vi "UI.vi"(0 "reference in":refnum<class "GUI Work Windows.lvclass">, 5 "error in (no error)":errorcluster) -> (14 "reference out":refnum<class "GUI Work Windows.lvclass">, 19 "error out":errorcluster)   [LabVIEW 2019, in "GUI Work Windows.lvclass"]
uses:
  GUI Work Windows.lvclass
  D:/GIT H4000/H4000/src/GUI_class/GUI.lvclass
  TypeDef/Data Stand.ctl
  TypeDef/Mode.ctl
  TypeDef/ExecuteStepState.ctl
  TypeDef/Direction.ctl
  Modbus_class/STS REG.ctl
  TypeDef/SP_TYPE.ctl
  TypeDef/State 44-1-2.ctl
  Modbus_class/CMD REG.ctl
  GUI_class/GUI.lvclass/GUI.ctl
  TypeDef/AI_Data_Array.ctl
  TypeDef/AI_Data.ctl
  TypeDef/AI Statistics Data.ctl
  FPGA/TypeDef/AI index.ctl
  SV_Wrap/SharedVariableWrapper.lvclass/SharedVariableWrapper.ctl
  Logger_class/Current Alarms.ctl
  Logger_class/EventData.ctl
  TypeDef/AlarmType.ctl
  MessageAMC_class/MessageAMC.lvclass
  D:/GIT H4000/H4000/src/MessageInterface_class/MessageInterface.lvclass
  f117a657-4c7e-47d8-9c03-ebf14d957611.vi
  1dd7af2e-2118-4c7c-a33f-1a736c63832f.vi
  8ac79095-62ac-4481-ab6e-8384228cdb70.vi
  41a135e7-8ee8-4611-b48a-c3c60048d180.vi
  6e9eca7a-d5d6-4f73-afb0-1afe8d30e139.vi
  a088a5f2-3759-4c3f-ba66-888ae32085c6.vi
  020c85a8-0765-46a5-946e-679e8cc30ba7.vi
  a65858e0-b92e-4e89-be62-7fc9634f1b2d.vi
  b775c166-e071-486c-b96e-0b96b0641e47.vi
  bf4e41d3-c56e-4c10-8d22-db1e327fdeb2.vi
  f5c6e87b-12af-4f11-98e9-46c3725dc062.vi
  c40ac8ee-f23a-4eac-9387-617ed5b7c06a.vi
  4e247ec6-9307-4091-8dab-29632f0d07b9.vi
  6be4fd1c-314b-4f5a-9423-f44751c79fde.vi
  010ce43b-0ee2-4248-bca4-f765867da5e8.vi
  GUI_class/Set Win State.vi
  GUI_class/protected/GetSheredData.vi
  8ac79095-62ac-4481-ab6e-8384228cdb70.vi/e1ff1487-cd56-43d2-a3a5-d033708db06e.vi
  SV_Wrap/Write Var Info.vi
  SV_Wrap/Read Var Info.vi
  41a135e7-8ee8-4611-b48a-c3c60048d180.vi/1efd96e0-8378-4666-9377-02721ba78358.vi
  6e9eca7a-d5d6-4f73-afb0-1afe8d30e139.vi/bae99f4a-ec10-4ec0-96ec-6d26d63f25ad.vi
  a088a5f2-3759-4c3f-ba66-888ae32085c6.vi/8d9527f5-1861-4624-9257-997a85ef616e.vi
  020c85a8-0765-46a5-946e-679e8cc30ba7.vi/7d84ca54-f83c-4ce5-86c1-7a192ad6100d.vi
  a65858e0-b92e-4e89-be62-7fc9634f1b2d.vi/5b02730d-42c6-4a71-85e1-f046919fac21.vi
  SV_Wrap/Read connection str.vi
  <userlib>/_OpenG.lib/time/time.llb/Tick Count (ms)__ogtk.vi
  GUI_class/GUI.lvclass
  SV_Wrap/SharedVariableWrapper.lvclass
  MessageInterface_class/MessageInterface.lvclass
panel:
  in  "hold":bool caption="Разрешить удержание"
  out "duration":i64
  out "delta dut 2":dbl caption="Погрешность [%]" format="%.1g"
  out "delta dut":dbl caption="Погрешность [%]" format="%.1g"
  in  "buret time":u16 caption="Время открытия бюретки [сек]"
  in  "nitro":bool caption="Азот"
  in  "burette":bool caption="Бюретка"
  in  "sp chamber":dbl caption="Уставка камера [МПа]"
  in  "sp dut":dbl caption="Уставка образец [МПа]"
  in  "CMD REG":T1
  out "leak":dbl(graph) caption="Давление датчик утечек [МПа]"
  out "data out":T2={"CommCounter"=0, "BeginFilingLevel"=0.0, "SP DUT"=0.0, "SP CHAMBER"=0.0, "Mode"=enum."IDLE", "ExecuteStepState"=enum."Init", "Direction"=enum."DUT", "Direction Filling"=enum."DUT", "STS"={"IDLE"=FALSE, "RYADY"=FALSE, "STEP"=FALSE, "ALARM"=FALSE, "WARNING"=FALSE, "REMOTE"=FALSE, "SP_EXEC_DONE_DUT"=FALSE, "SP_EXEC_DONE_CHAMBER"=FALSE, "FILING_DONE_DUT"=FALSE, "FILING_DONE_CHAMBER"=FALSE, "BURETE_STATE"=FALSE}, "SP_TYPE_DUT"=enum."ZIRO", "SP_TYPE_CHAMBER"=enum."ZIRO", "New Step"=FALSE, "BURETE_TIME"=0, "With BURETE"=FALSE, "With Nitro"=FALSE, "State 44-1-2"=enum."Init", "Measure leak"=FALSE, "hold"=FALSE}
  in  "clear chart":bool
  in  "Multicolumn Listbox":i32(listbox)=-1
  out "error":bool caption="Подключение"
  out "chmbr":T9(graph) caption="Давление камера [МПа]"
  out "dut":T9(graph) caption="Давление образец [МПа]"
  in  "remote":bool caption="Разрешить внешнее управление"
  in  "stop":bool
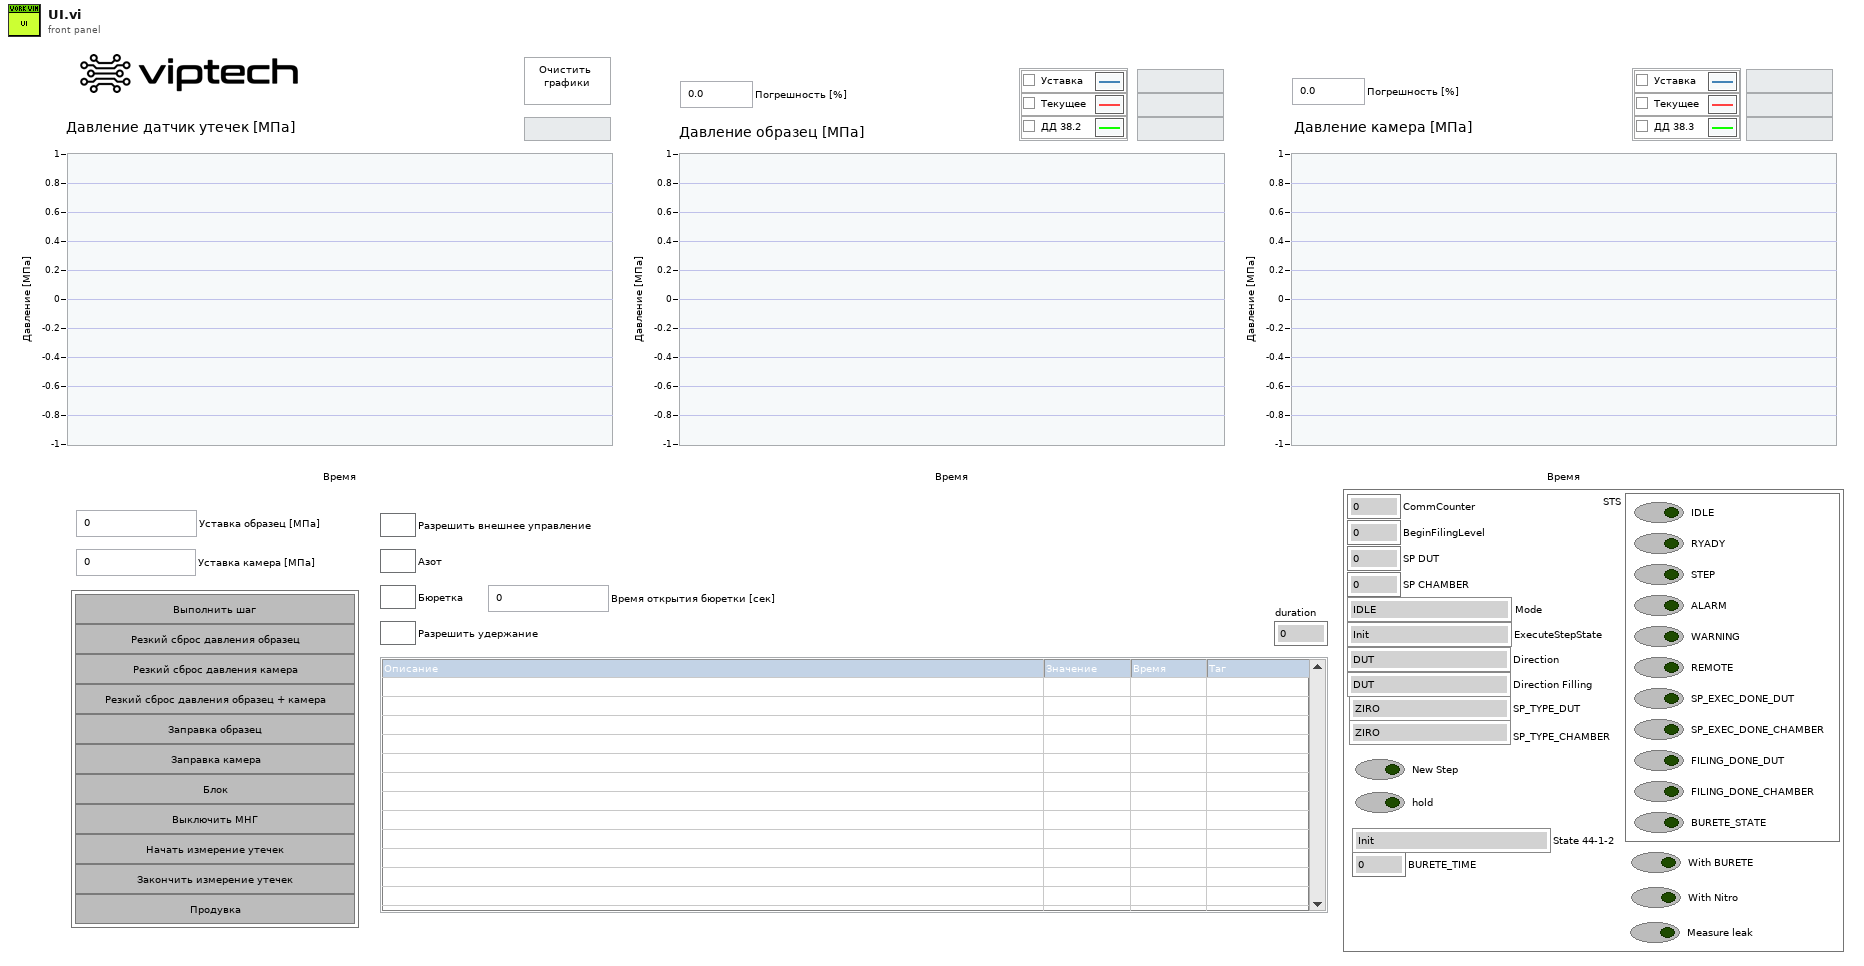
[diagram p1: front panel]
types:
  T1 = typedef "CMD REG.ctl" = cluster{"EXECUTE_SP":bool, "ALARM_PRESS_DOWN_DUT":bool, "ALARM_PRESS_DOWN_CHAMBER":bool, "ALARM_PRESS_DOWN_DUT_CHAMBER":bool, "FILING_DUT":bool, "FILING_CHAMBER":bool, "BLOCK":bool, "PUMP_STATION_OFF":bool, "Leak start":bool, "Leak stop":bool, "Drain":bool}
  T2 = typedef "Data Stand.ctl" = cluster{"CommCounter":u64, "BeginFilingLevel":dbl, "SP DUT":dbl, "SP CHAMBER":dbl, "Mode":T3, "ExecuteStepState":T4, "Direction":T5, "Direction Filling":T5, "STS":T6, "SP_TYPE_DUT":T7, "SP_TYPE_CHAMBER":T7, "New Step":bool, "BURETE_TIME":u16, "With BURETE":bool, "With Nitro":bool, "State 44-1-2":T8, "Measure leak":bool, "hold":bool}
  T3 = typedef "Mode.ctl" = enum16{"IDLE", "FILLING", "EXECUTE_SP", "DRAIN"}
  T4 = typedef "ExecuteStepState.ctl" = enum16{"Init", "Set: Backpressure ", "Preload: HI", "Set: HI", "Maintenance: HI", "Down: Pressure", "BLOCK"}
  T5 = typedef "Direction.ctl" = enum8{"DUT", "Chamber"}
  T6 = typedef "STS REG.ctl" = cluster{"IDLE":bool, "RYADY":bool, "STEP":bool, "ALARM":bool, "WARNING":bool, "REMOTE":bool, "SP_EXEC_DONE_DUT":bool, "SP_EXEC_DONE_CHAMBER":bool, "FILING_DONE_DUT":bool, "FILING_DONE_CHAMBER":bool, "BURETE_STATE":bool}
  T7 = typedef "SP_TYPE.ctl" = enum16{"ERROR", "ZIRO", "BASE", "SP"}
  T8 = typedef "State 44-1-2.ctl" = enum16{"Init", "Idle", "Wait", "Open 44-1", "Open 44-2", "Close 44-1", "Close 44-2"}
  T9 = cluster{"Pressure SP":dbl, "scl mean 1Hz":dbl, "scl mean 1Hz":dbl}
  T10 = enum32{"Invalid", "Standard", "Closed", "Hidden", "Minimized", "Maximized"}
  T11 = enum32{"invalid app kind", "Development System", "Run Time System", "Student Edition", "Embedded LabVIEW", "Evaluation", "Custom"}
  T12 = typedef "SharedVariableWrapper.lvclass/Config.ctl" = cluster{"connection str":string, "timeout":dbl, "ip":string}
  T13 = cluster{"Core":cluster{"Current VI Reference":refnum<vi>, "Close Panel on Exit?":bool}, "amc":refnum<class "MessageAMC.lvclass">}
  T14 = cluster{"Current VI Reference":refnum<vi>, "Close Panel on Exit?":bool}
  T15 = typedef "AI_Data_Array.ctl" = T16[]
  T16 = typedef "AI_Data.ctl" = cluster{"Stat Data":T17, "OutOfRangeMax":bool, "OutOfRangeMin":bool, "HIHI":bool, "HI":bool, "LO":bool, "LOLO":bool}
  T17 = typedef "AI Statistics Data.ctl" = cluster{"raw mean":dbl, "scl mean":dbl, "raw mean 1Hz":dbl, "scl mean 1Hz":dbl}
  T18 = typedef "Current Alarms.ctl" = cluster{"alarms":T19[]}
  T19 = typedef "EventData.ctl" = cluster{"obj_tag":string, "event_tag":string, "Description":string, "ALARM TYPE":T20, "Value DBL":dbl, "Value INT":i32, "Value STR":string, "Time Stamp":timestamp}
  T20 = typedef "AlarmType.ctl" = enum16{"Normal", "Warning", "Alarm"}
  T21 = typedef "AI index.ctl" = u8
  T22 = cluster{"SP DUT":dbl, "scl mean 1Hz":dbl, "scl mean 1Hz":dbl}
  T23 = cluster{"SP CHAMBER":dbl, "scl mean 1Hz":dbl, "scl mean 1Hz":dbl}
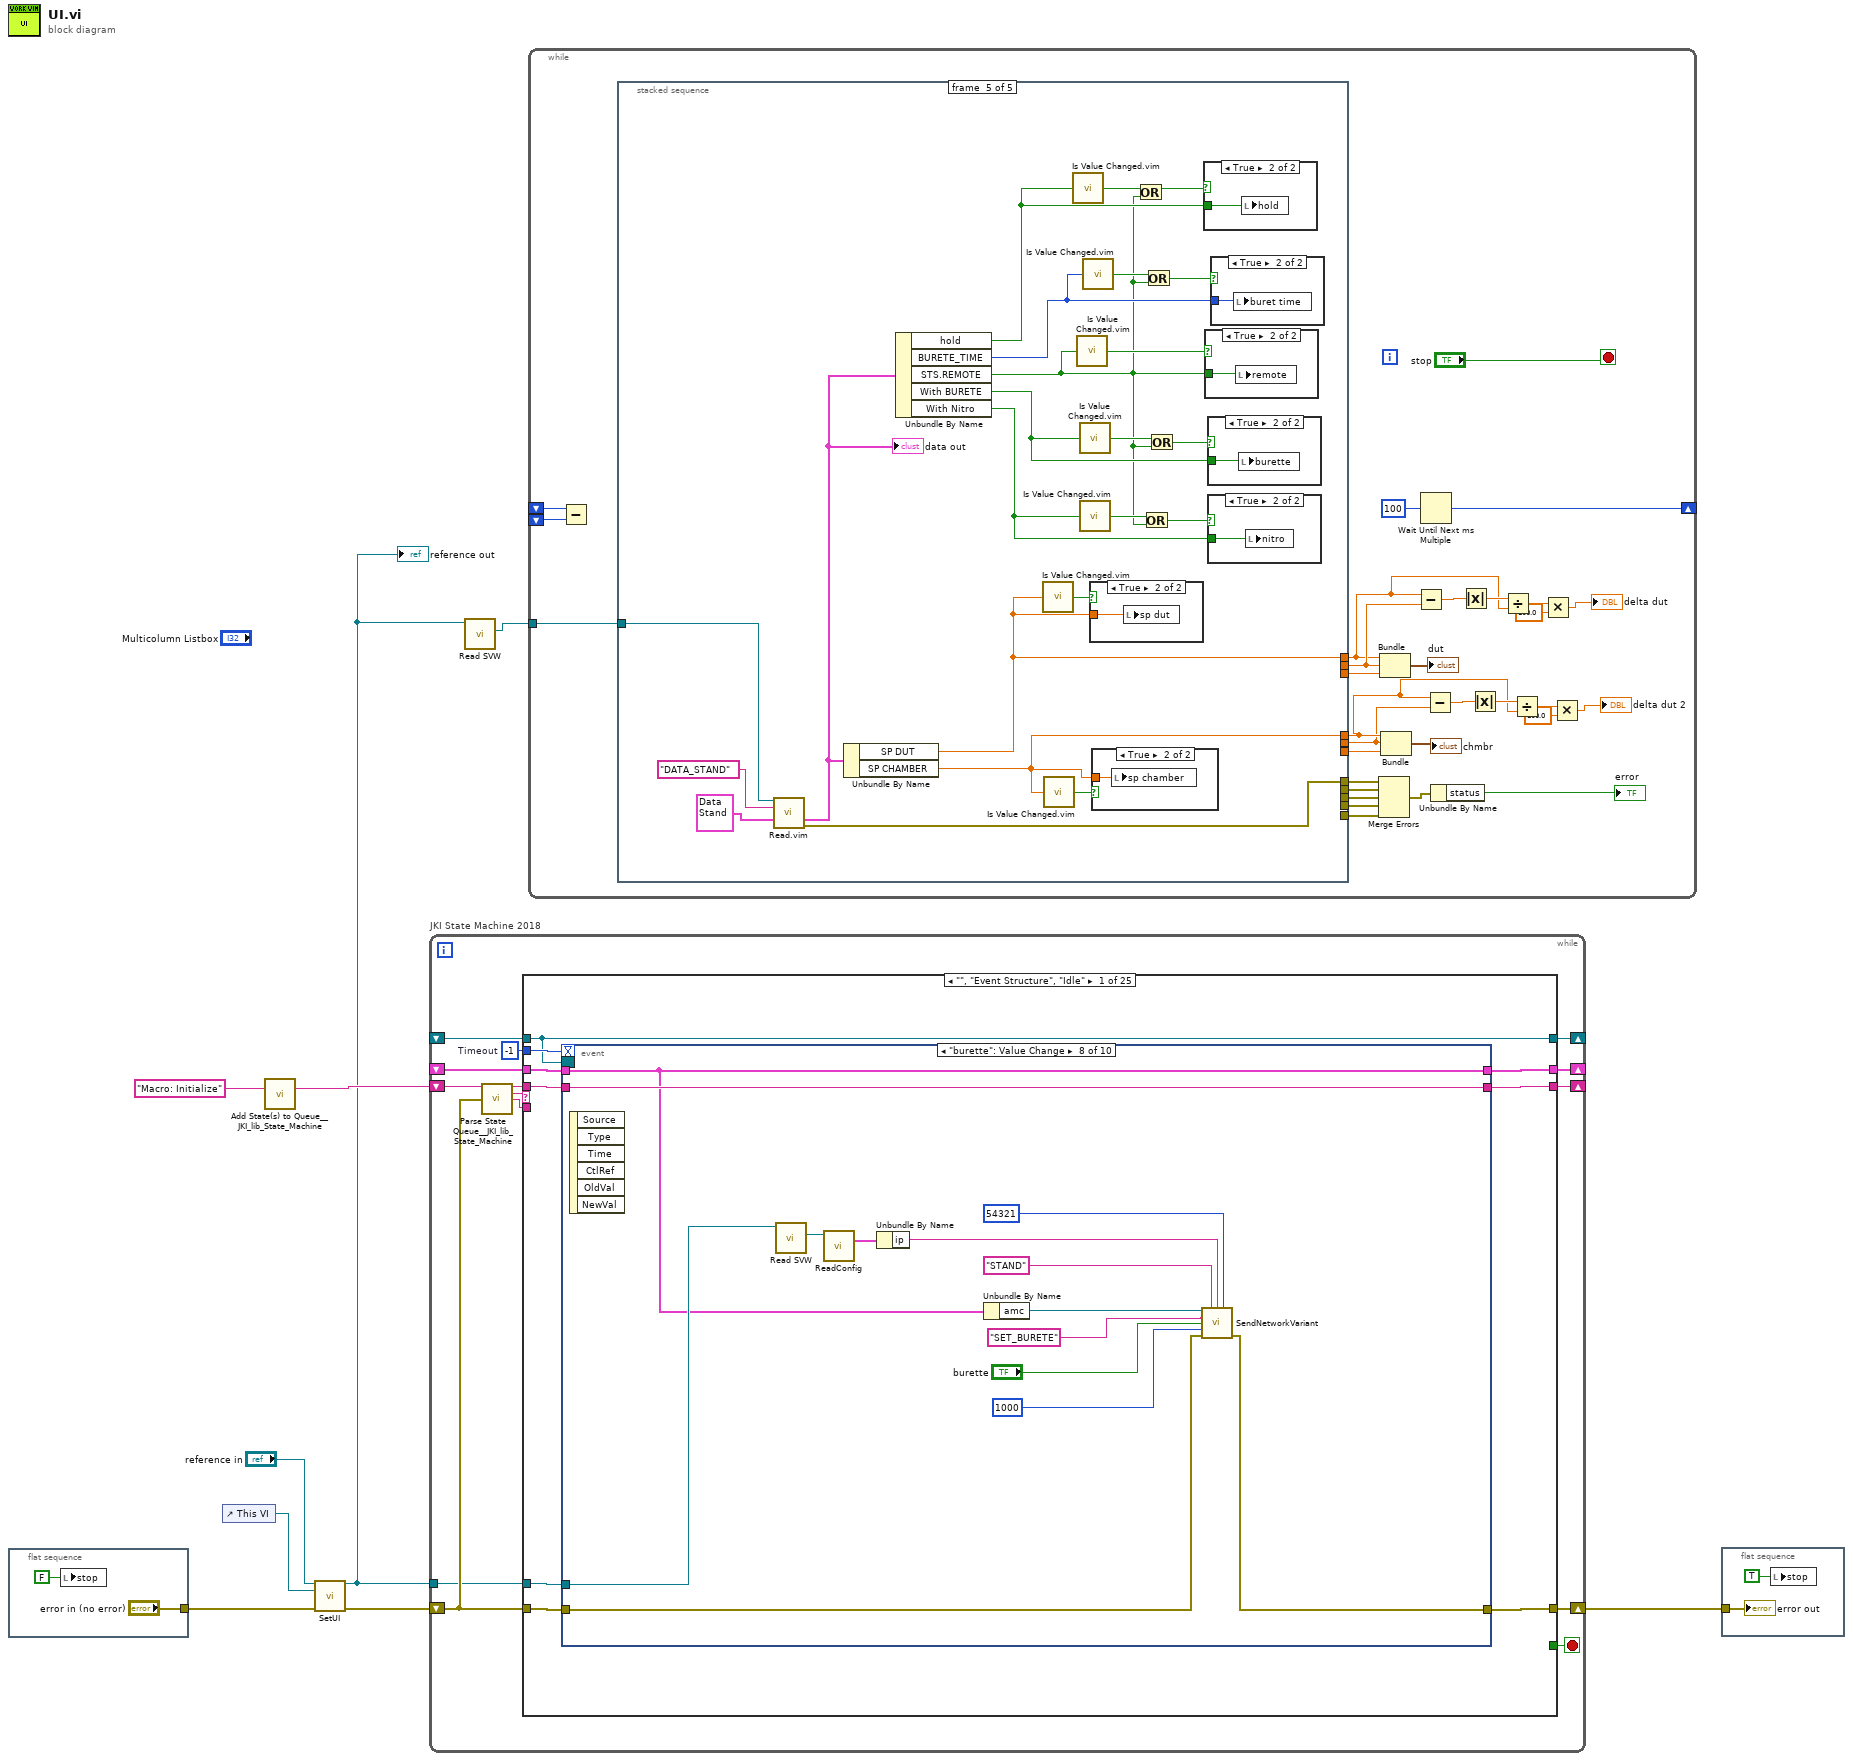
[diagram p0: block diagram]
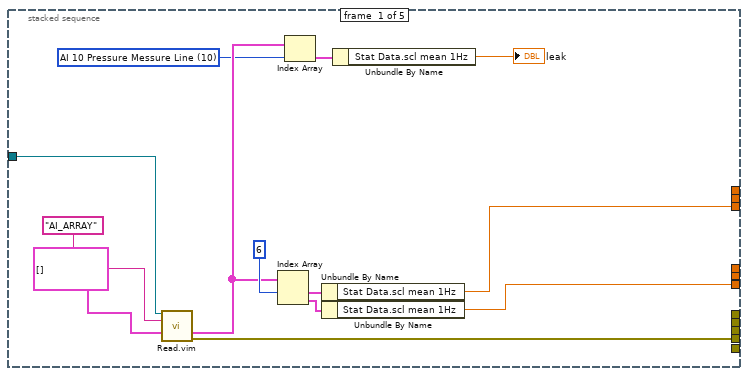
[diagram p2: hidden frame]
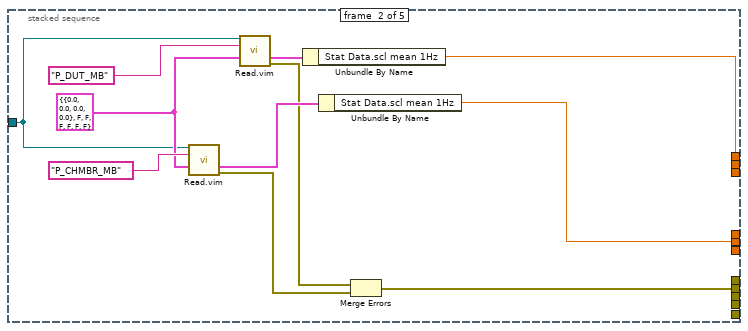
[diagram p3: hidden frame]
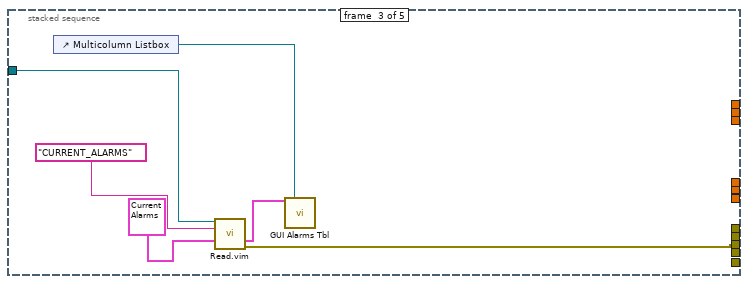
[diagram p4: hidden frame]
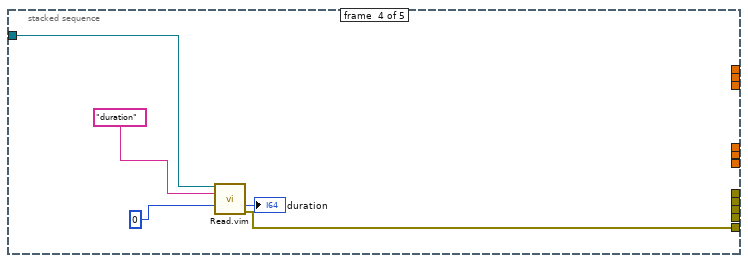
[diagram p5: hidden frame]
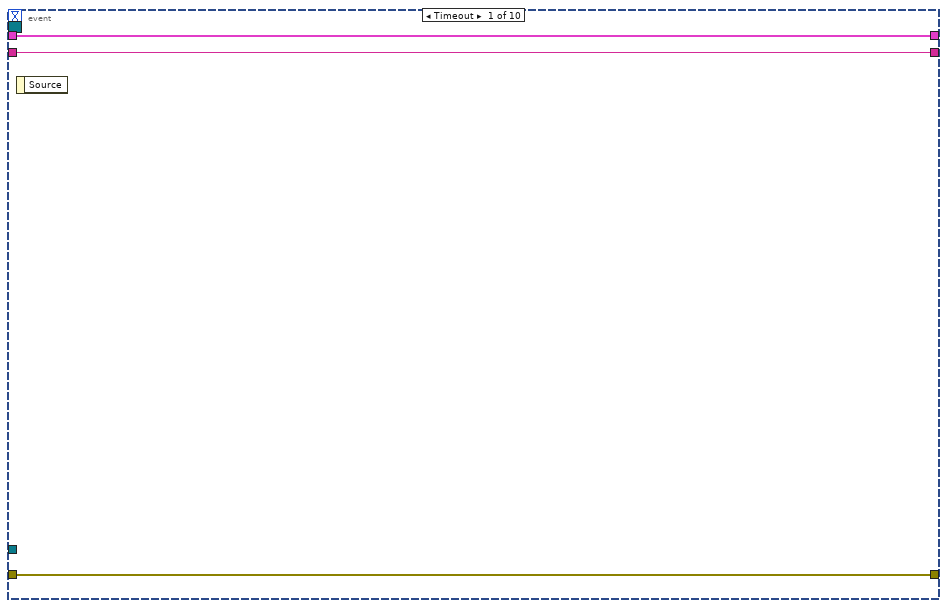
[diagram p13: hidden frame]
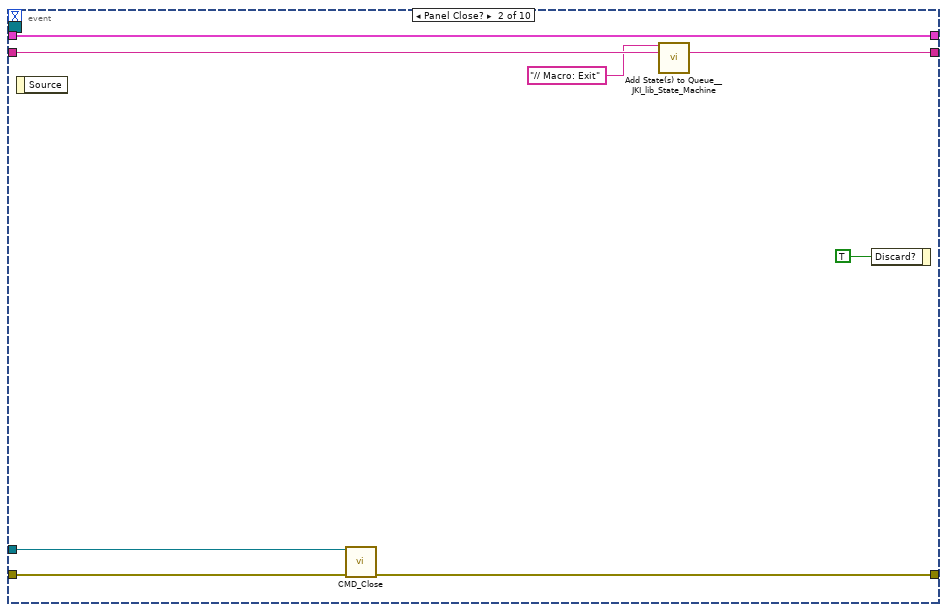
[diagram p14: hidden frame]
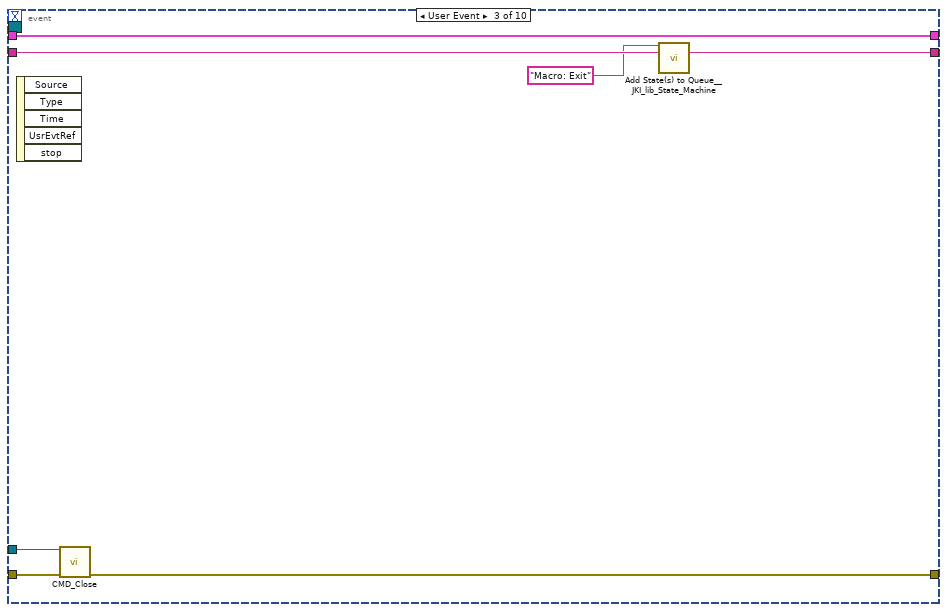
[diagram p15: hidden frame]
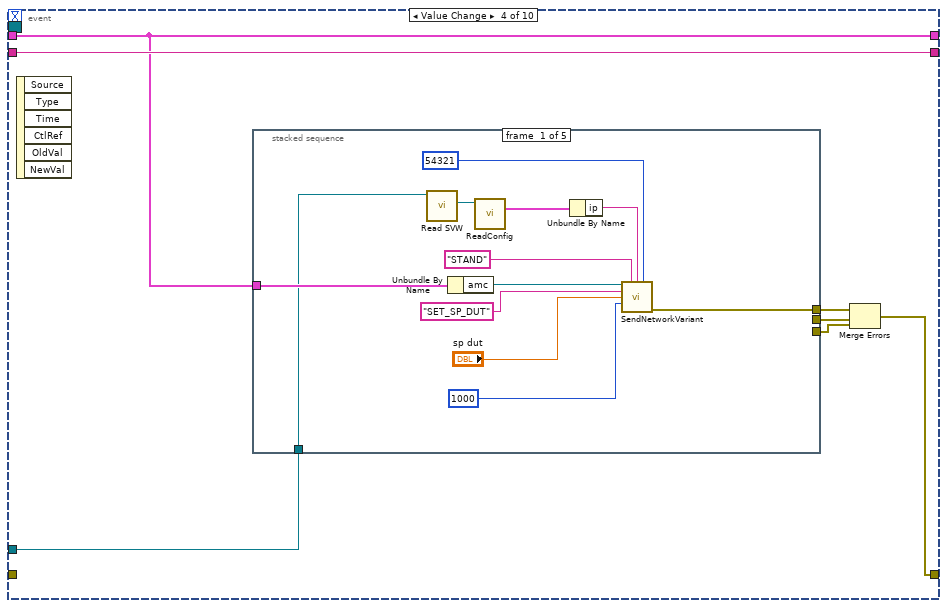
[diagram p16: hidden frame]
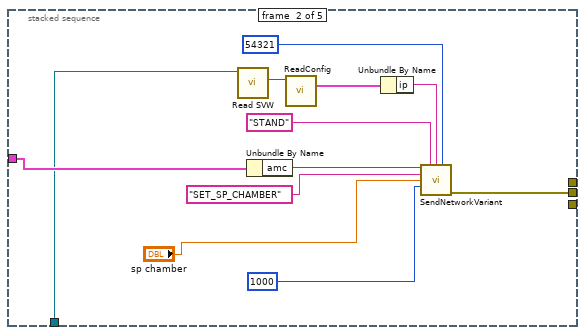
[diagram p17: hidden frame]
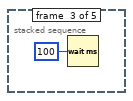
[diagram p18: hidden frame]
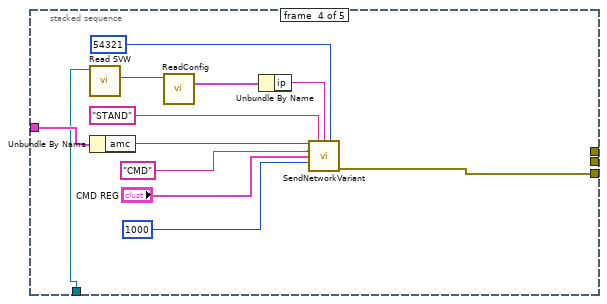
[diagram p19: hidden frame]
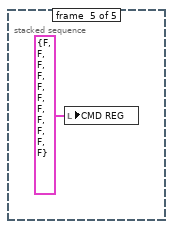
[diagram p20: hidden frame]
diagram:
  n1 = flat-sequence {
    tunnel: ["error in (no error)"] -> w6
    frame #0 {
      n2 = local write "stop"(FALSE ("stop")) -> ()
    }
  }
  n3 = control-ref of="This VI"() -> (w4:refnum<vi>)
  n4 = call <vilib>:"Add State(s) to Queue__JKI_lib_State_Machine.vi"("State(s) in (\"\")"="Macro: Initialize") -> ("States Out"=w9:string)  [unwired: 14 in]
  n5 = call "SetUI.vi"("reference in"="reference in", "UI VI"=w4, "error in (no error)"=w6) -> ("reference out"=w2:refnum<class "GUI Work Windows.lvclass">, "error out"=w3:errorcluster)  [unwired: 11 in]
  "reference out" <- w2
  n6 = while "JKI State Machine 2018" {
    shift-right: [w18] -> _
    shift-left: _ -> [w17]
    shift-right: [w21] -> w7
    shift-left: w3 -> [w15]
    shift-right: [w20] -> _
    shift-left: w9 -> [w22]
    tunnel: w2 -> [w14]
    shift-right: [w13] -> _
    shift-left: _ -> [w12]
    stop <- w19 stop-if-true
    w16 = -1  # Timeout
    n7 = call <vilib>:"Parse State Queue__JKI_lib_State_Machine.vi"("State Queue"=w22, "Error In (no error)"=w15) -> ("Remaining States"=w24:string, "Current State"=w25:string, "Arguments"=w23:string)  [unwired: 11 in]
    n8 = case shown="\"\", \"Event Structure\", \"Idle\"" w25 {
      selector: w25 -> [_ _ w186 _ _ _ _ _ _ _ _ _ _ _ _ _ _ _ _ _ _ _ _ _ _]
      tunnel: w24 -> [w34 w184 w190 w210 w217 w225 w230 w239 w246 w251 w258 w264 w269 w273 w280 w292 w362 w368 w374 w386 w390 w391 w400 w404 w406]
      tunnel: w23 -> [_ _ _ _ _ _ _ _ _ _ _ _ _ _ w275 w286 _ _ _ _ _ _ _ _ _]
      tunnel: w17 -> [w32 w181 w188 w203 w214 w220 w227 _ w241 w248 w257 w262 w266 w272 w278 w288 w359 w365 w371 w383 w388 w393 w398 w401 w405]
      tunnel: [w31 w182 w192 w207 errorcluster {"status"=FALSE, "code"=0, "source"=""} ("error out") w223 w228 w232 w242 w249 w255 w259 w267 w271 w276 w289 w360 w366 w372 w384 w389 w394 w397 w402 w408] -> w21
      tunnel: w15 -> [w30 w182 w191 w207 w213 w223 w228 w233 w243 w249 w254 w260 w267 w271 w277 w290 w360 w366 w372 w384 w389 w394 w397 w402 w408]
      tunnel: [w33 w183 w189 w209 w216 w224 w229 w239 w245 w250 w258 w263 w268 w273 w279 w291 w361 w367 w373 w385 w390 w392 w400 w404 w406] -> w20
      tunnel: [_ _ _ _ _ TRUE _ _ _ _ _ _ _ _ _ _ _ _ _ _ _ _ _ _ _] -> w19
      tunnel: [w29 w181 w188 w208 w214 w220 w227 w238 w241 w248 w257 w262 w266 w272 w278 w288 w359 w365 w371 w383 w388 w393 w398 w401 w405] -> w18
      tunnel: w16 -> [w28 _ _ _ _ _ _ _ _ _ _ _ _ _ _ _ _ _ _ _ _ _ _ _ _]
      tunnel: w14 -> [w27 _ _ _ _ _ _ _ _ _ w253 _ _ _ _ _ _ _ _ _ _ w395 _ _ _]
      tunnel: [w26 w180 w185 w197 w211 w221 w226 w236 w240 w247 w256 w261 w265 w270 w274 w285 w358 w363 w369 w376 w387 w396 w399 w403 w407] -> w13
      tunnel: w12 -> [w26 w180 w185 w197 w211 w221 w226 w236 w240 w247 _ w261 w265 w270 w274 w285 w358 w363 w369 w376 w387 w396 w399 w403 w407]
      frame "", "Event Structure", "Idle" {
        n9 = event shown="[7] \"burette\": Value Change" {
          selector: w26 -> [_ _ _ _ _ _ _ _ _ _]
          dyn-events: _ -> [_ _ _ _ _ _ _ _ _ _]
          timeout: w28 -> [_ _ _ _ _ _ _ _ _ _]
          tunnel: w34 -> [w37 w45 w52 w59 w106 w123 w137 w151 w165 w179]
          tunnel: [w37 w44 w51 w59 w106 w123 w137 w151 w165 w179] -> w33
          tunnel: w32 -> [w35 w43 w50 w58 w105 w118 w132 w146 w160 w174]
          tunnel: [w36 w38 w46 w53 w99 w111 w125 w139 w153 w167] -> w31
          tunnel: w30 -> [w36 w39 w47 _ w104 w112 w126 w140 w154 w168]
          tunnel: [w35 w43 w50 w58 w105 w118 w132 w146 w160 w174] -> w29
          tunnel: w27 -> [_ w40 w48 w57 _ w119 w133 w147 w161 w175]
          event Timeout {
            n10 = event-data() -> ()  [unwired: 1 in, 1 out]
          }
          event Panel Close? {
            n11 = event-data() -> ()  [unwired: 1 in, 1 out]
            n12 = call "CMD_Close.vi"("reference in"=w40, "error in (no error)"=w39) -> ("error out"=w38:errorcluster)  [unwired: 12 in, 1 out]
            n13 = call <vilib>:"Add State(s) to Queue__JKI_lib_State_Machine.vi"("State(s) in Front (\"\")"="// Macro: Exit", "State(s) in (\"\")"=w45) -> ("States Out"=w44:string)  [unwired: 13 in]
            n14 = event-data("Discard?"=TRUE) -> ()  [unwired: 1 in, 1 out]
          }
          event User Event {
            n15 = event-data() -> ()  [unwired: 1 in, 5 out]
            n16 = call "CMD_Close.vi"("reference in"=w48, "error in (no error)"=w47) -> ("error out"=w46:errorcluster)  [unwired: 12 in, 1 out]
            n17 = call <vilib>:"Add State(s) to Queue__JKI_lib_State_Machine.vi"("State(s) in Front (\"\")"="Macro: Exit", "State(s) in (\"\")"=w52) -> ("States Out"=w51:string)  [unwired: 13 in]
          }
          event Value Change {
            n18 = event-data() -> ()  [unwired: 1 in, 6 out]
            n19 = stacked-sequence {
              tunnel: w58 -> [w63 w74 _ w87 _]
              tunnel: w57 -> [w62 w73 _ w85 _]
              tunnel: [w61 _ _ _ _] -> w54
              tunnel: [_ w72 _ _ _] -> w55
              tunnel: [_ _ _ w88 _] -> w56
              frame #0 {
                n20 = call "Read SVW.vi"("GUI in"=w62) -> ("SharedVariableWrapper.lvclass"=w68:refnum<class "SharedVariableWrapper.lvclass">)  [unwired: 10 in]
                n21 = Unbundle By Name(w63) -> ("amc"=w60:refnum<class "MessageAMC.lvclass">)
                n22 = call "ReadConfig.vi"("SharedVariableWrapper in"=w68) -> ("config"=w69:T12)  [unwired: 12 in, 2 out]
                n23 = Unbundle By Name(w69) -> ("ip"=w70:string)
                n24 = call "SendNetworkVariant.vi"("reference in"=w60, "receiver process"="STAND", "receiver host"=w70, "receiver port (0)"=u16 54321, "name"="SET_SP_DUT", "data"="sp dut", "timeout (25000 ms)"=1000) -> ("error out"=w61:errorcluster)  [unwired: 6 in, 2 out]
              }
              frame #1 {
                n25 = call "Read SVW.vi"("GUI in"=w73) -> ("SharedVariableWrapper.lvclass"=w79:refnum<class "SharedVariableWrapper.lvclass">)  [unwired: 10 in]
                n26 = Unbundle By Name(w74) -> ("amc"=w82:refnum<class "MessageAMC.lvclass">)
                n27 = call "ReadConfig.vi"("SharedVariableWrapper in"=w79) -> ("config"=w80:T12)  [unwired: 12 in, 2 out]
                n28 = Unbundle By Name(w80) -> ("ip"=w81:string)
                n29 = call "SendNetworkVariant.vi"("reference in"=w82, "receiver process"="STAND", "receiver host"=w81, "receiver port (0)"=u16 54321, "name"="SET_SP_CHAMBER", "data"="sp chamber", "timeout (25000 ms)"=1000) -> ("error out"=w72:errorcluster)  [unwired: 6 in, 2 out]
              }
              frame #2 {
                n30 = Wait (ms)(milliseconds to wait=u32 100) -> ()  [unwired: 1 out]
              }
              frame #3 {
                n31 = call "Read SVW.vi"("GUI in"=w85) -> ("SharedVariableWrapper.lvclass"=w96:refnum<class "SharedVariableWrapper.lvclass">)  [unwired: 10 in]
                n32 = Unbundle By Name(w87) -> ("amc"=w86:refnum<class "MessageAMC.lvclass">)
                n33 = call "ReadConfig.vi"("SharedVariableWrapper in"=w96) -> ("config"=w95:T12)  [unwired: 12 in, 2 out]
                n34 = Unbundle By Name(w95) -> ("ip"=w94:string)
                n35 = call "SendNetworkVariant.vi"("reference in"=w86, "receiver process"="STAND", "receiver host"=w94, "receiver port (0)"=u16 54321, "name"="CMD", "data"="CMD REG", "timeout (25000 ms)"=1000) -> ("error out"=w88:errorcluster)  [unwired: 6 in, 2 out]
              }
              frame #4 {
                n36 = local write "CMD REG"(T1 {"EXECUTE_SP"=FALSE, "ALARM_PRESS_DOWN_DUT"=FALSE, "ALARM_PRESS_DOWN_CHAMBER"=FALSE, "ALARM_PRESS_DOWN_DUT_CHAMBER"=FALSE, "FILING_DUT"=FALSE, "FILING_CHAMBER"=FALSE, "BLOCK"=FALSE, "PUMP_STATION_OFF"=FALSE, "Leak start"=FALSE, "Leak stop"=FALSE, "Drain"=FALSE} ("CMD REG")) -> ()
              }
            }
            n37 = Merge Errors(w54, w55, w56) -> (w53:errorcluster)
          }
          event "clear chart": Value Change {
            n38 = event-data() -> ()  [unwired: 1 in, 6 out]
            n39 = control-ref of="dut"() -> (w103:refnum<vi>)
            n40 = control-ref of="chmbr"() -> (w102:refnum<vi>)
            n41 = Build Array(w103, w102) -> (w101:refnum<vi>[])
            n42 = control-ref of="leak"() -> (w98:refnum<vi>)
            n43 = for {
              shift-right: [w108] -> w100
              shift-left: w104 -> [w109]
              tunnel: w101 -> [w107] mode=indexing
              n44 = call "Waveform Clear Hist.vim"("error in (no error)"=w109, "WaveformChart in"=w107) -> ("error out"=w108:errorcluster)  [unwired: 9 in]
            }
            n45 = call "Waveform Clear Hist.vim"("error in (no error)"=w100, "WaveformChart in"=w98) -> ("error out"=w99:errorcluster)  [unwired: 9 in]
          }
          event "remote": Value Change {
            n46 = event-data() -> ()  [unwired: 1 in, 6 out]
            n47 = call "Read SVW.vi"("GUI in"=w119) -> ("SharedVariableWrapper.lvclass"=w122:refnum<class "SharedVariableWrapper.lvclass">)  [unwired: 10 in]
            n48 = call "ReadConfig.vi"("SharedVariableWrapper in"=w122) -> ("config"=w121:T12)  [unwired: 12 in, 2 out]
            n49 = Unbundle By Name(w121) -> ("ip"=w120:string)
            n50 = Unbundle By Name(w118) -> ("amc"=w117:refnum<class "MessageAMC.lvclass">)
            n51 = call "SendNetworkVariant.vi"("reference in"=w117, "receiver process"="STAND", "receiver host"=w120, "receiver port (0)"=u16 54321, "name"="SET_REMOTE", "data"="remote", "timeout (25000 ms)"=1000, "error in (no error)"=w112) -> ("error out"=w111:errorcluster)  [unwired: 5 in, 2 out]
          }
          event "hold": Value Change {
            n52 = event-data() -> ()  [unwired: 1 in, 6 out]
            n53 = call "Read SVW.vi"("GUI in"=w133) -> ("SharedVariableWrapper.lvclass"=w136:refnum<class "SharedVariableWrapper.lvclass">)  [unwired: 10 in]
            n54 = call "ReadConfig.vi"("SharedVariableWrapper in"=w136) -> ("config"=w135:T12)  [unwired: 12 in, 2 out]
            n55 = Unbundle By Name(w135) -> ("ip"=w134:string)
            n56 = Unbundle By Name(w132) -> ("amc"=w131:refnum<class "MessageAMC.lvclass">)
            n57 = call "SendNetworkVariant.vi"("reference in"=w131, "receiver process"="STAND", "receiver host"=w134, "receiver port (0)"=u16 54321, "name"="SET_HOLD", "data"="hold", "timeout (25000 ms)"=1000, "error in (no error)"=w126) -> ("error out"=w125:errorcluster)  [unwired: 5 in, 2 out]
          }
          event "burette": Value Change {
            n58 = event-data() -> ()  [unwired: 1 in, 6 out]
            n59 = call "Read SVW.vi"("GUI in"=w147) -> ("SharedVariableWrapper.lvclass"=w150:refnum<class "SharedVariableWrapper.lvclass">)  [unwired: 10 in]
            n60 = call "ReadConfig.vi"("SharedVariableWrapper in"=w150) -> ("config"=w149:T12)  [unwired: 12 in, 2 out]
            n61 = Unbundle By Name(w149) -> ("ip"=w148:string)
            n62 = Unbundle By Name(w146) -> ("amc"=w145:refnum<class "MessageAMC.lvclass">)
            n63 = call "SendNetworkVariant.vi"("reference in"=w145, "receiver process"="STAND", "receiver host"=w148, "receiver port (0)"=u16 54321, "name"="SET_BURETE", "data"="burette", "timeout (25000 ms)"=1000, "error in (no error)"=w140) -> ("error out"=w139:errorcluster)  [unwired: 5 in, 2 out]
          }
          event "nitro": Value Change {
            n64 = event-data() -> ()  [unwired: 1 in, 6 out]
            n65 = call "Read SVW.vi"("GUI in"=w161) -> ("SharedVariableWrapper.lvclass"=w164:refnum<class "SharedVariableWrapper.lvclass">)  [unwired: 10 in]
            n66 = call "ReadConfig.vi"("SharedVariableWrapper in"=w164) -> ("config"=w163:T12)  [unwired: 12 in, 2 out]
            n67 = Unbundle By Name(w163) -> ("ip"=w162:string)
            n68 = Unbundle By Name(w160) -> ("amc"=w159:refnum<class "MessageAMC.lvclass">)
            n69 = call "SendNetworkVariant.vi"("reference in"=w159, "receiver process"="STAND", "receiver host"=w162, "receiver port (0)"=u16 54321, "name"="SET_NITRO", "data"="nitro", "timeout (25000 ms)"=1000, "error in (no error)"=w154) -> ("error out"=w153:errorcluster)  [unwired: 5 in, 2 out]
          }
          event "buret time": Value Change {
            n70 = event-data() -> ()  [unwired: 1 in, 6 out]
            n71 = call "Read SVW.vi"("GUI in"=w175) -> ("SharedVariableWrapper.lvclass"=w178:refnum<class "SharedVariableWrapper.lvclass">)  [unwired: 10 in]
            n72 = call "ReadConfig.vi"("SharedVariableWrapper in"=w178) -> ("config"=w177:T12)  [unwired: 12 in, 2 out]
            n73 = Unbundle By Name(w177) -> ("ip"=w176:string)
            n74 = Unbundle By Name(w174) -> ("amc"=w173:refnum<class "MessageAMC.lvclass">)
            n75 = call "SendNetworkVariant.vi"("reference in"=w173, "receiver process"="STAND", "receiver host"=w176, "receiver port (0)"=u16 54321, "name"="SET_BURETE_TIME", "data"="buret time", "timeout (25000 ms)"=1000, "error in (no error)"=w168) -> ("error out"=w167:errorcluster)  [unwired: 5 in, 2 out]
          }
        }
      }
      frame "---------- Core ----------" {
        n76 = call <vilib>:"Add State(s) to Queue__JKI_lib_State_Machine.vi"("State(s) in (\"\")"=w184) -> ("States Out"=w183:string)  [unwired: 14 in]
      }
      frame Default {
        w195 = 42 items=["No error", "Argument error", "Memory is full", "Out of zone", "End of file", "File already open", "Generic file I/O error", "File not found", "File permission error", "Disk is full", "Duplicate path", "Too many files open", "System feature not enabled", "Resource file not found", "Cannot add resource", "Resource not found", "Image not found", "Image memory error", "Pen does not exist", "Config type invalid", "Config token not found", "Config parse error", "Config memory error", "Bad external code format", "Bad external code offset", "External code not present", "Null window", "Destroy window error", "Null menu", "Print aborted", "Bad print record", "Print driver error", "Windows error during printing", "Memory error during printing", "Print dialog error", "Generic print error", "Invalid device refnum", "Device not found", "Device parameter error", "Device unit error", "Cannot open device", "Device call aborted", "Generic error", "Cancelled by user", "Object ID too low", "Object ID too high", "Object not in heap", "Unknown heap", "Unknown object (invalid DefProc)", "Unknown object (DefProc not in table)", "Message out of range", "Invalid (null) method", "Unknown message", "Manager call not supported", "Bad address", "Network operation in progress", "Network operation timed out", "Connection is busy", "Network attribute not supported", "Network error", "Address in use", "System out of memory", "Connection aborted", "Connection refused", "Not connected", "Already connected", "Connection closed", "Initialization error (interapplication manager)", "Bad occurrence", "Wait on unbound occurrence handler", "Occurrence queue overflow", "Datalog type conflict", "Unused", "Unrecognized type (interapplication manager)", "Memory corrupt", "Failed to make temporary DLL", "Old CIN version", "Drag socket not found", "Failed to load drop-object", "Failed to register OLE object", "Failed to release OLE object", "Format specifier type mismatch", "Unknown format specifier", "Too few format specifiers", "Too many format specifiers", "Scan failed", "Newer CIN version", "Error converting to variant", "Runtime menu error", "Password tampered", "Variant attribute not found", "Incompatible variant data type", "Event data is not available", "Event Store is not present", "Occurrence is not found", "Event Queue is not created", "Event info is not available", "Refnum passed is NULL", "Error retrieving Class GUID", "Error retrieving CoClass GUID", "Error retrieving TypeLib GUID.", "Bad built application magic bytes.", "Specific driver is different from the specific driver associated with the Logical Name.", "There is no session opened to the class driver.", "Max Error", "MAX - Error with config objects", "MAX - Error loading configuration", "MAX - Group not supported"]
        # "Current State"
        # "Do not delete, rename, or modify this frame.\n(this is used to capture unhandled states and typos)"
        # "Handle mistyped state name (developer tool)"
        n77 = Format Into String(format string="Software Exception: Unhandled State \"%s\"." ("message"), error in=w191, w186) -> (resulting string=w194:string, error out=w193:errorcluster)  [unwired: 1 in]
        n78 = call <vilib>:"Error Cluster From Error Code.vi"("show call chain? (False)"=TRUE, "error in (no error)"=w193, "error message (\"\")"=w194, "error code (0)"=w195) -> ("error out"=w192:errorcluster)  [unwired: 5 in]
        n79 = call <vilib>:"Add State(s) to Queue__JKI_lib_State_Machine.vi"("State(s) in (\"\")"=w190) -> ("States Out"=w189:string)  [unwired: 14 in]
      }
      frame "Initialize Core Data" {
        # "Do not delete, rename, or modify this frame.\n(this is used to determine panel behavior on exit)"
        # "originally closed?"
        # "exe?"
        # "If panel starts closed or is an EXE, then close it when we exit"
        n80 = property class="VI"() -> ("FP.State"=w200:T10)  [unwired: 2 in, 2 out]
        n81 = property class="App"() -> ("App.Kind"=w206:T11)  [unwired: 2 in, 2 out]
        n82 = control-ref of="Current VI Reference"() -> (w201:refnum<vi>)
        n83 = Equal?(x=w200, y=T10."Closed" ("Front Panel Window:State")) -> (x = y?=w198:bool)
        n84 = Equal?(x=w206, y=T11."Run Time System" ("Application:Kind")) -> (x = y?=w204:bool)
        n85 = Or(x=w198, y=w204) -> (x .or. y?=w202:bool)
        n86 = Bundle By Name(cluster=w203, "Core.Current VI Reference"=w201, "Core.Close Panel on Exit?"=w202) -> (w208:T13)
        n87 = call <vilib>:"Add State(s) to Queue__JKI_lib_State_Machine.vi"("State(s) in (\"\")"=w210) -> ("States Out"=w209:string)  [unwired: 14 in]
      }
      frame "Error Handler" {
        # "Unhandled Error -- Display it"
        # "Handle any errors here.\nYou can also output any states to clean-up after errors occur"
        # "Clear error"
        n88 = call <vilib>:"General Error Handler.vi"("error in (no error)"=w213) -> ()  [unwired: 10 in, 5 out]
        n89 = call <vilib>:"Add State(s) to Queue__JKI_lib_State_Machine.vi"("State(s) in Front (\"\")"="/* Post Error States", "State(s) in (\"\")"=w217) -> ("States Out"=w216:string)  [unwired: 13 in]
      }
      frame "Exit" {
        n90 = Unbundle By Name(w220) -> ("amc"=w219:refnum<class "MessageAMC.lvclass">)
        n91 = call-dynamic "Destroy.vi"("reference in"=w219) -> ("error out"=w218:errorcluster)  [unwired: 17 in, 1 out]
        n92 = call <vilib>:"Clear Errors.vi"("error in (no error)"=w218) -> ()  [unwired: 5 in, 2 out]
        n93 = call <vilib>:"Add State(s) to Queue__JKI_lib_State_Machine.vi"("State(s) in (\"\")"=w225) -> ("States Out"=w224:string)  [unwired: 14 in]
      }
      frame "---------- Data ----------" {
        # "Do not put any code in this frame.\n(It is a separator no-op. You can make a copy of this frame to create a new Data frame)"
        n94 = call <vilib>:"Add State(s) to Queue__JKI_lib_State_Machine.vi"("State(s) in (\"\")"=w230) -> ("States Out"=w229:string)  [unwired: 14 in]
      }
      frame "Data: Initialize" {
        w237 = T14 {"Current VI Reference"=refnum, "Close Panel on Exit?"=FALSE}  # Core
        n95 = call "MessageAMC_Create.vi"("reference in"=refnum<class "MessageAMC.lvclass"> refnum, "error in (no error)"=w233, "message queue name"="GUI_TEST_CHNLS") -> ("amc"=w234:refnum<class "MessageAMC.lvclass">, "error out"=w232:errorcluster)  [unwired: 15 in]
        n96 = Bundle("Core"=w237, "amc"=w234) -> (w238:T13)  [unwired: 1 in]
      }
      frame "Data: Cleanup" {
        # "Cleanup any data and references, here.\n(this is called automatically, by the Macro: Exit)"
        n97 = Unbundle By Name(w241) -> ("Core.Current VI Reference"=w244:refnum<vi>)
        n98 = Close Reference(reference=w244, error in (no error)=w243) -> (error out=w242:errorcluster)
        n99 = call <vilib>:"Add State(s) to Queue__JKI_lib_State_Machine.vi"("State(s) in (\"\")"=w246) -> ("States Out"=w245:string)  [unwired: 14 in]
      }
      frame "---------- Events ----------" {
        # "Do not put any code in this frame.\n(It is a separator no-op. You can make a copy of this frame to create a new UI frame)"
        n100 = call <vilib>:"Add State(s) to Queue__JKI_lib_State_Machine.vi"("State(s) in (\"\")"=w251) -> ("States Out"=w250:string)  [unwired: 14 in]
      }
      frame "Events: Register" {
        n101 = call "Read stop event.vi"("GUI in"=w253) -> ("stop event"=w252:refnum<user-event>)  [unwired: 8 in, 2 out]
        n102 = register-events(error in=w254, w252) -> (reference out=w256:refnum<event-registration>, error out=w255:errorcluster)  [unwired: 1 in]
      }
      frame "Events: Unregister" {
        # "Do not put any code in this frame.\n(It is a separator no-op. You can make a copy of this frame to create a new UI frame)"
        n103 = Unregister For Events(event registration refnum=w261, error in=w260) -> (error out=w259:errorcluster)
        n104 = call <vilib>:"Add State(s) to Queue__JKI_lib_State_Machine.vi"("State(s) in (\"\")"=w264) -> ("States Out"=w263:string)  [unwired: 14 in]
      }
      frame "---------- UI ----------" {
        # "Do not put any code in this frame.\n(It is a separator no-op. You can make a copy of this frame to create a new UI frame)"
        n105 = call <vilib>:"Add State(s) to Queue__JKI_lib_State_Machine.vi"("State(s) in (\"\")"=w269) -> ("States Out"=w268:string)  [unwired: 14 in]
      }
      frame "UI: Initialize" {
      }
      frame "UI: Cursor Set" {
        # "Argument"
        # "Set and Unset Cursor Busy.\n(Usage: \"UI: Cursor Set >> Busy|Idle\")"
        n106 = case shown="\"Idle\", Default" w275 {
          tunnel: w277 -> [w282 w284]
          tunnel: [w281 w283] -> w276
          frame "Idle", Default {
            n107 = call <vilib>:"Unset Busy.vi"("error in (no error)"=w282) -> ("error out"=w281:errorcluster)  [unwired: 10 in]
          }
          frame "Busy" {
            n108 = call <vilib>:"Set Busy.vi"("error in (no error)"=w284) -> ("error out"=w283:errorcluster)  [unwired: 9 in, 1 out]
          }
        }
        n109 = call <vilib>:"Add State(s) to Queue__JKI_lib_State_Machine.vi"("State(s) in (\"\")"=w280) -> ("States Out"=w279:string)  [unwired: 14 in]
      }
      frame "UI: Front Panel State" {
        # "Argument"
        # "Set Front Panel Open or Closed\n(Usage: \"UI: Front Panel State >> Open|Close\")"
        n110 = Unbundle By Name(w288) -> ("Core.Current VI Reference"=w287:refnum<vi>)
        n111 = case shown="\"Minimize\", \"Minimized\"" w286 {
          tunnel: w290 -> [w298 w313 w324 w337 w350]
          tunnel: [w300 w314 w326 w339 w352] -> w289
          tunnel: w287 -> [w299 w311 w325 w338 w351]
          frame "Open", "Standard", Default {
            w293 = T10."Standard" ("State")
            n112 = property class="VI"(reference=w299, error in=w298) -> (reference out=w296:refnum<vi>, error out=w297:errorcluster, "FP.State"=w295:T10)
            n113 = Not Equal?(x=w295, y=w293) -> (x != y?=w294:bool)
            n114 = case shown="True" w294 {
              tunnel: [w304 w306] -> w300
              tunnel: w297 -> [w303 w306]
              tunnel: w296 -> [w302 _]
              tunnel: w293 -> [w301 _]
              frame True {
                n115 = invoke class="VI" method="FP.Open"(reference=w302, error in=w303, "Activate"=TRUE, "State"=w301) -> (error out=w304:errorcluster)  [unwired: 1 in, 4 out]
              }
              frame False {
              }
            }
          }
          frame "Close", "Closed" {
            n116 = property class="VI"(reference=w311, error in=w313) -> (reference out=w310:refnum<vi>, error out=w312:errorcluster, "FP.State"=w308:T10)
            n117 = Not Equal?(x=w308, y=T10."Closed" ("Front Panel Window:State")) -> (x != y?=w307:bool)
            n118 = case shown="True" w307 {
              tunnel: [w315 w318] -> w314
              tunnel: w312 -> [w315 w317]
              tunnel: w310 -> [_ w316]
              frame False {
              }
              frame True {
                n119 = invoke class="VI" method="FP.Close"(reference=w316, error in=w317) -> (error out=w318:errorcluster)  [unwired: 1 in, 2 out]
              }
            }
          }
          frame "Hidden", "Hide" {
            w319 = T10."Hidden" ("State")
            n120 = property class="VI"(reference=w325, error in=w324) -> (reference out=w322:refnum<vi>, error out=w323:errorcluster, "FP.State"=w321:T10)
            n121 = Not Equal?(x=w321, y=w319) -> (x != y?=w320:bool)
            n122 = case shown="True" w320 {
              tunnel: [w330 w331] -> w326
              tunnel: w323 -> [w329 w331]
              tunnel: w322 -> [w328 _]
              tunnel: w319 -> [w327 _]
              frame True {
                n123 = invoke class="VI" method="FP.Open"(reference=w328, error in=w329, "State"=w327) -> (error out=w330:errorcluster)  [unwired: 2 in, 4 out]
              }
              frame False {
              }
            }
          }
          frame "Minimize", "Minimized" {
            w332 = T10."Minimized" ("State")
            n124 = property class="VI"(reference=w338, error in=w337) -> (reference out=w335:refnum<vi>, error out=w336:errorcluster, "FP.State"=w334:T10)
            n125 = Not Equal?(x=w334, y=w332) -> (x != y?=w333:bool)
            n126 = case shown="True" w333 {
              tunnel: [w343 w344] -> w339
              tunnel: w336 -> [w342 w344]
              tunnel: w335 -> [w341 _]
              tunnel: w332 -> [w340 _]
              frame True {
                n127 = invoke class="VI" method="FP.Open"(reference=w341, error in=w342, "State"=w340) -> (error out=w343:errorcluster)  [unwired: 2 in, 4 out]
              }
              frame False {
              }
            }
          }
          frame "Maximize", "Maximized" {
            w345 = T10."Maximized" ("State")
            n128 = property class="VI"(reference=w351, error in=w350) -> (reference out=w348:refnum<vi>, error out=w349:errorcluster, "FP.State"=w347:T10)
            n129 = Not Equal?(x=w347, y=w345) -> (x != y?=w346:bool)
            n130 = case shown="True" w346 {
              tunnel: [w356 w357] -> w352
              tunnel: w349 -> [w355 w357]
              tunnel: w348 -> [w354 _]
              tunnel: w345 -> [w353 _]
              frame True {
                n131 = invoke class="VI" method="FP.Open"(reference=w354, error in=w355, "State"=w353) -> (error out=w356:errorcluster)  [unwired: 2 in, 4 out]
              }
              frame False {
              }
            }
          }
        }
        n132 = call <vilib>:"Add State(s) to Queue__JKI_lib_State_Machine.vi"("State(s) in (\"\")"=w292) -> ("States Out"=w291:string)  [unwired: 14 in]
      }
      frame "---------- Macro ----------" {
        # "Do not put any code in this frame.\n(It is a separator no-op. You can make a copy of this frame to create a new Macro frame)"
        n133 = call <vilib>:"Add State(s) to Queue__JKI_lib_State_Machine.vi"("State(s) in (\"\")"=w362) -> ("States Out"=w361:string)  [unwired: 14 in]
      }
      frame "Macro: Initialize" {
        n134 = call <vilib>:"Add State(s) to Queue__JKI_lib_State_Machine.vi"("State(s) in Front (\"\")"="Data: Initialize\nInitialize Core Data\nEvents: Register\nUI: Initialize\n// UI: Front Panel State >> Open\n\n\nAction: Read Config\nAction: Update Indicators\n", "State(s) in (\"\")"=w368) -> ("States Out"=w367:string)  [unwired: 13 in]
      }
      frame "Macro: Update" {
        n135 = call <vilib>:"Add State(s) to Queue__JKI_lib_State_Machine.vi"("State(s) in Front (\"\")"="Action: Update Indicators\nAction: Write Config", "State(s) in (\"\")"=w374) -> ("States Out"=w373:string)  [unwired: 13 in]
      }
      frame "Macro: Exit" {
        # "Exit Macro\n(This is called once, when the VI exits)"
        n136 = Unbundle By Name(w383) -> ("Core.Close Panel on Exit?"=w382:bool)
        n137 = Select(t="UI: Front Panel State >> Close", s=w382, f="") -> (s? t:f=w379:string)
        n138 = call <vilib>:"Add State(s) to Queue__JKI_lib_State_Machine.vi"("State(s) in Front (\"\")"="Action: Write Config", "State(s) in (\"\")"=w379, "State(s) at Back (\"\")"="Data: Cleanup\nEvents: Unregister\nExit") -> ("States Out"=w377:string)  [unwired: 12 in]
        n139 = call <vilib>:"Add State(s) to Queue__JKI_lib_State_Machine.vi"("State(s) in Front (\"\")"=w377, "State(s) in (\"\")"=w386) -> ("States Out"=w385:string)  [unwired: 13 in]
      }
      frame "---------- Action ----------" {
      }
      frame "Action: Read Config" {
        n140 = call "Read ConfigInterface.vi"("GUI in"=w395) -> ()  [unwired: 9 in, 2 out]
        n141 = call <vilib>:"Add State(s) to Queue__JKI_lib_State_Machine.vi"("State(s) in (\"\")"=w391) -> ("States Out"=w392:string)  [unwired: 14 in]
      }
      frame "Action: Write Config" {
      }
      frame "Action: Update Indicators" {
      }
      frame "Action: Update Channels TBL" {
      }
    }
  }
  n142 = call "Read SVW.vi"("GUI in"=w2) -> ("SharedVariableWrapper.lvclass"=w1:refnum<class "SharedVariableWrapper.lvclass">)  [unwired: 10 in]
  n143 = while {
    tunnel: w1 -> [w439]
    shift-right: [w436] -> _
    shift-left: _ -> [w435]
    shift-left: _ -> [w434]
    stop <- "stop" stop-if-true
    n144 = Subtract(x=w435, y=w434) -> ()  [unwired: 1 out]
    n145 = stacked-sequence {
      tunnel: w439 -> [w448 w458 w467 w473 w494]
      tunnel: [_ _ w466 _ _] -> w433
      tunnel: [w447 _ _ _ _] -> w432
      tunnel: [w446 _ _ _ _] -> w431
      tunnel: [_ w457 _ _ _] -> w423
      tunnel: [_ w456 _ _ _] -> w410
      tunnel: [w445 _ _ _ _] -> w428
      tunnel: [_ w454 _ _ _] -> w427
      tunnel: [_ _ _ _ w488] -> w426
      tunnel: [_ _ _ _ w491] -> w420
      tunnel: [_ _ _ _ w489] -> w411
      tunnel: [_ _ _ w472 _] -> w409
      frame #0 {
        w443 = T21 10 items=["AI 0 Cooling Station Level", "AI 1 Cooling Station Temp", "AI 2 Oil Supply Level", "AI 3 Oil Supply Temp", "AI 4 ", "AI 5 Pressure Haskel", "AI 6 Pressure DUT", "AI 7 Pressure Chamber", "AI 8 Pressure Air inlet", "AI 9 Pressure Air outlet", "AI 10 Pressure Messure Line", "AI 11 DUT 2", "AI 12 Chamber 2"] ("AI index")
        n146 = call "Read.vim"("SharedVariableWrapper in"=w448, "name"="AI_ARRAY", "DataType"=T15 [] ("AI_Data_Array")) -> ("data out"=w444:T15, "error out"=w445:errorcluster)  [unwired: 6 in, 5 out]
        n147 = Index Array(array=w444, index #1=6 ("index")) -> (element #1=w440:T16, element #2=w449:T16)  [unwired: 1 in]
        n148 = Index Array(array=w444, index=w443) -> (element=w442:T16)
        n149 = Unbundle By Name(w440) -> ("Stat Data.scl mean 1Hz"=w447:dbl)
        n150 = Unbundle By Name(w449) -> ("Stat Data.scl mean 1Hz"=w446:dbl)
        n151 = Unbundle By Name(w442) -> ("Stat Data.scl mean 1Hz"=→"leak":dbl)
      }
      frame #1 {
        w461 = T16 {"Stat Data"={"raw mean"=0.0, "scl mean"=0.0, "raw mean 1Hz"=0.0, "scl mean 1Hz"=0.0}, "OutOfRangeMax"=FALSE, "OutOfRangeMin"=FALSE, "HIHI"=FALSE, "HI"=FALSE, "LO"=FALSE, "LOLO"=FALSE} ("AI_Data")
        n152 = call "Read.vim"("SharedVariableWrapper in"=w458, "name"="P_CHMBR_MB", "DataType"=w461) -> ("data out"=w459:T16, "error out"=w453:errorcluster)  [unwired: 6 in, 5 out]
        n153 = call "Read.vim"("SharedVariableWrapper in"=w458, "name"="P_DUT_MB", "DataType"=w461) -> ("data out"=w460:T16, "error out"=w455:errorcluster)  [unwired: 6 in, 5 out]
        n154 = Unbundle By Name(w460) -> ("Stat Data.scl mean 1Hz"=w457:dbl)
        n155 = Unbundle By Name(w459) -> ("Stat Data.scl mean 1Hz"=w456:dbl)
        n156 = Merge Errors(w455, w453) -> (w454:errorcluster)
      }
      frame #2 {
        n157 = control-ref of="Multicolumn Listbox"() -> (w464:refnum<vi>)
        n158 = call "Read.vim"("SharedVariableWrapper in"=w467, "name"="CURRENT_ALARMS", "DataType"=T18 {"alarms"=[{"obj_tag"="AI0", "event_tag"="AI0.OUT_OF_RANGE_MIN", "Description"="Уровень  масла (НС очистки и охлаждения). Вне диапазона (низкий уровень)", "ALARM TYPE"=enum."Alarm", "Value DBL"=0.0, "Value INT"=1, "Value STR"="Alarm", "Time Stamp"=timestamp(3830845009.237916 s since 1904-01-01)}, {"obj_tag"="AI1", "event_tag"="AI1.OUT_OF_RANGE_MIN", "Description"="Уровень масла (НС подачи масла). Вне диапазона (низкий уровень)", "ALARM TYPE"=enum."Alarm", "Value DBL"=0.0, "Value INT"=1, "Value STR"="Alarm", "Time Stamp"=timestamp(3830845009.237916 s since 1904-01-01)}, {"obj_tag"="AI10", "event_tag"="AI10.OUT_OF_RANGE_MIN", "Description"="Датчик давления в линии измерения утечек. Вне диапазона (низкий уровень)", "ALARM TYPE"=enum."Alarm", "Value DBL"=0.0, "Value INT"=1, "Value STR"="Alarm", "Time Stamp"=timestamp(3830845009.237916 s since 1904-01-01)}, {"obj_tag"="AI2", "event_tag"="AI2.OUT_OF_RANGE_MIN", "Description"="Температура масла (НС очистки и охлаждения). Вне диапазона (низкий уровень)", "ALARM TYPE"=enum."Alarm", "Value DBL"=0.0, "Value INT"=1, "Value STR"="Alarm", "Time Stamp"=timestamp(3830845009.237916 s since 1904-01-01)}, {"obj_tag"="AI3", "event_tag"="AI3.OUT_OF_RANGE_MIN", "Description"="Температура масла (НС подачи масла). Вне диапазона (низкий уровень)", "ALARM TYPE"=enum."Alarm", "Value DBL"=0.0, "Value INT"=1, "Value STR"="Alarm", "Time Stamp"=timestamp(3830845009.237916 s since 1904-01-01)}, {"obj_tag"="AI4", "event_tag"="AI4.OUT_OF_RANGE_MIN", "Description"="Обратная связь от клапана регулировки низкого давления . Вне диапазона (низкий уровень)", "ALARM TYPE"=enum."Alarm", "Value DBL"=0.0, "Value INT"=1, "Value STR"="Alarm", "Time Stamp"=timestamp(3830845009.237916 s since 1904-01-01)}, {"obj_tag"="AI5", "event_tag"="AI5.OUT_OF_RANGE_MIN", "Description"="Давление после насоса ВД. Вне диапазона (низкий уровень)", "ALARM TYPE"=enum."Alarm", "Value DBL"=0.0, "Value INT"=1, "Value STR"="Alarm", "Time Stamp"=timestamp(3830845009.237916 s since 1904-01-01)}, {"obj_tag"="AI6", "event_tag"="AI6.OUT_OF_RANGE_MIN", "Description"="Давление в образце. Вне диапазона (низкий уровень)", "ALARM TYPE"=enum."Alarm", "Value DBL"=0.0, "Value INT"=1, "Value STR"="Alarm", "Time Stamp"=timestamp(3830845009.237916 s since 1904-01-01)}, {"obj_tag"="AI7", "event_tag"="AI7.OUT_OF_RANGE_MIN", "Description"="Давление в камере. Вне диапазона (низкий уровень)", "ALARM TYPE"=enum."Alarm", "Value DBL"=0.0, "Value INT"=1, "Value STR"="Alarm", "Time Stamp"=timestamp(3830845009.237916 s since 1904-01-01)}, {"obj_tag"="AI8", "event_tag"="AI8.OUT_OF_RANGE_MIN", "Description"="Давление  в  линии подачи воздуха в  БПВ. Вне диапазона (низкий уровень)", "ALARM TYPE"=enum."Alarm", "Value DBL"=0.0, "Value INT"=1, "Value STR"="Alarm", "Time Stamp"=timestamp(3830845009.237916 s since 1904-01-01)}, {"obj_tag"="AI9", "event_tag"="AI9.OUT_OF_RANGE_MIN", "Description"="Давление  в  линии подачи воздуха после БПВ. Вне диапазона (низкий уровень)", "ALARM TYPE"=enum."Alarm", "Value DBL"=0.0, "Value INT"=1, "Value STR"="Alarm", "Time Stamp"=timestamp(3830845009.237916 s since 1904-01-01)}, {"obj_tag"="M12", "event_tag"="M12.AUTOMAT_ERROR", "Description"="Двигатель перекачки. Выключен автомат", "ALARM TYPE"=enum."Alarm", "Value DBL"=1.0, "Value INT"=1, "Value STR"="Alarm", "Time Stamp"=timestamp(3830845009.739716 s since 1904-01-01)}, {"obj_tag"="M21", "event_tag"="M21.AUTOMAT_ERROR", "Description"="Двигатель подачи масла. Выключен автомат", "ALARM TYPE"=enum."Alarm", "Value DBL"=1.0, "Value INT"=1, "Value STR"="Alarm", "Time Stamp"=timestamp(3830845009.739716 s since 1904-01-01)}, {"obj_tag"="M22", "event_tag"="M22.AUTOMAT_ERROR", "Description"="Двигатель охлаждения. Выключен автомат", "ALARM TYPE"=enum."Alarm", "Value DBL"=1.0, "Value INT"=1, "Value STR"="Alarm", "Time Stamp"=timestamp(3830845009.739716 s since 1904-01-01)}]} ("data in")) -> ("data out"=w465:T18, "error out"=w466:errorcluster)  [unwired: 6 in, 5 out]
        n159 = call "GUI Alarms Tbl.vi"("data in"=w465, "Multicolumn Listbox ref"=w464) -> ()  [unwired: 12 in, 2 out]
      }
      frame #3 {
        n160 = call "Read.vim"("SharedVariableWrapper in"=w473, "name"="duration", "DataType"=i64 0) -> ("data out"=→"duration":i64, "error out"=w472:errorcluster)  [unwired: 6 in, 5 out]
      }
      frame #4 {
        n161 = call "Read.vim"("SharedVariableWrapper in"=w494, "name"="DATA_STAND", "DataType"=T2 {"CommCounter"=0, "BeginFilingLevel"=0.0, "SP DUT"=0.0, "SP CHAMBER"=0.0, "Mode"=enum."IDLE", "ExecuteStepState"=enum."Init", "Direction"=enum."DUT", "Direction Filling"=enum."DUT", "STS"={"IDLE"=FALSE, "RYADY"=FALSE, "STEP"=FALSE, "ALARM"=FALSE, "WARNING"=FALSE, "REMOTE"=FALSE, "SP_EXEC_DONE_DUT"=FALSE, "SP_EXEC_DONE_CHAMBER"=FALSE, "FILING_DONE_DUT"=FALSE, "FILING_DONE_CHAMBER"=FALSE, "BURETE_STATE"=FALSE}, "SP_TYPE_DUT"=enum."ZIRO", "SP_TYPE_CHAMBER"=enum."ZIRO", "New Step"=FALSE, "BURETE_TIME"=0, "With BURETE"=FALSE, "With Nitro"=FALSE, "State 44-1-2"=enum."Init", "Measure leak"=FALSE, "hold"=FALSE} ("Data Stand")) -> ("data out"=w493:T2, "error out"=w488:errorcluster)  [unwired: 6 in, 5 out]
        "data out" <- w493
        n162 = Unbundle By Name(w493) -> ("SP DUT"=w491:dbl, "SP CHAMBER"=w489:dbl)
        n163 = Unbundle By Name(w493) -> ("hold"=w478:bool, "BURETE_TIME"=w482:u16, "STS.REMOTE"=w475:bool, "With BURETE"=w485:bool, "With Nitro"=w484:bool)
        n164 = call "Is Value Changed.vim"("value"=w491) -> ("changed or first call?"=w490:bool)
        n165 = call "Is Value Changed.vim"("value"=w489) -> ("changed or first call?"=w497:bool)
        n166 = call "Is Value Changed.vim"("value"=w478) -> ("changed or first call?"=w477:bool)
        n167 = call "Is Value Changed.vim"("value"=w475) -> ("changed or first call?"=w492:bool)
        n168 = call "Is Value Changed.vim"("value"=w485) -> ("changed or first call?"=w487:bool)
        n169 = call "Is Value Changed.vim"("value"=w484) -> ("changed or first call?"=w486:bool)
        n170 = call "Is Value Changed.vim"("value"=w482) -> ("changed or first call?"=w483:bool)
        n171 = case shown="True" w490 {
          tunnel: w491 -> [_ w502]
          frame False {
          }
          frame True {
            n172 = local write "sp dut"(w502) -> ()
          }
        }
        n173 = case shown="True" w497 {
          tunnel: w489 -> [_ w504]
          frame False {
          }
          frame True {
            n174 = local write "sp chamber"(w504) -> ()
          }
        }
        n175 = Or(x=w477, y=w475) -> (x .or. y?=w476:bool)
        n176 = Or(x=w486, y=w475) -> (x .or. y?=w479:bool)
        n177 = Or(x=w483, y=w475) -> (x .or. y?=w481:bool)
        n178 = Or(x=w487, y=w475) -> (x .or. y?=w480:bool)
        n179 = case shown="True" w476 {
          tunnel: w478 -> [_ w498]
          frame False {
          }
          frame True {
            n180 = local write "hold"(w498) -> ()
          }
        }
        n181 = case shown="True" w492 {
          tunnel: w475 -> [_ w503]
          frame False {
          }
          frame True {
            n182 = local write "remote"(w503) -> ()
          }
        }
        n183 = case shown="True" w480 {
          tunnel: w485 -> [_ w501]
          frame False {
          }
          frame True {
            n184 = local write "burette"(w501) -> ()
          }
        }
        n185 = case shown="True" w479 {
          tunnel: w484 -> [_ w500]
          frame False {
          }
          frame True {
            n186 = local write "nitro"(w500) -> ()
          }
        }
        n187 = case shown="True" w481 {
          tunnel: w482 -> [_ w499]
          frame False {
          }
          frame True {
            n188 = local write "buret time"(w499) -> ()
          }
        }
      }
    }
    n189 = Merge Errors(w426, w427, w433, w428, w409) -> (w438:errorcluster)
    n190 = Bundle("SP DUT"=w420, "scl mean 1Hz"=w423, "scl mean 1Hz"=w432) -> (→"dut":T22)  [unwired: 1 in]
    n191 = Bundle("SP CHAMBER"=w411, "scl mean 1Hz"=w410, "scl mean 1Hz"=w431) -> (→"chmbr":T23)  [unwired: 1 in]
    n192 = Subtract(x=w420, y=w423) -> (x-y=w422:dbl)
    n193 = Wait Until Next ms Multiple(millisecond multiple=u32 100) -> (millisecond timer value=w436:u32)
    n194 = Subtract(x=w411, y=w410) -> (x-y=w412:dbl)
    n195 = Unbundle By Name(w438) -> ("status"=→"error":bool)
    n196 = Absolute Value(x=w422) -> (abs(x)=w421:dbl)
    n197 = Absolute Value(x=w412) -> (abs(x)=w413:dbl)
    n198 = Divide(x=w421, y=w420) -> (x/y=w419:dbl)
    n199 = Divide(x=w413, y=w411) -> (x/y=w414:dbl)
    n200 = Multiply(x=w419, y=100.0) -> (x*y=→"delta dut":dbl)
    n201 = Multiply(x=w414, y=100.0) -> (x*y=→"delta dut 2":dbl)
  }
  n202 = flat-sequence {
    tunnel: w7 -> [w506]
    frame #0 {
      n203 = local write "stop"(TRUE ("stop")) -> ()
      "error out" <- w506
    }
  }
